vi "Write Scale Fit.vi"(5 "Scale Fit":u8, 9 "GraphScale in":refnum<class "GraphScale.lvclass">) -> (3 "GraphScale out":refnum<class "GraphScale.lvclass">)   [LabVIEW 2014, in "GraphScale.lvclass"]
uses:
  GraphScale.lvclass
  GraphScale.lvclass/GraphScale.ctl
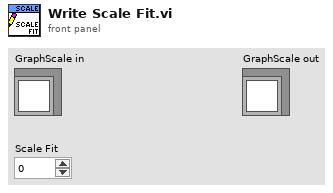
[diagram p1: front panel]
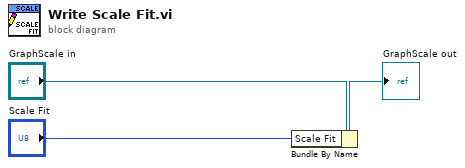
[diagram p0: block diagram]
diagram:
  n1 = Bundle By Name(cluster="GraphScale in", "Scale Fit"="Scale Fit") -> (→"GraphScale out":refnum<class "GraphScale.lvclass">)
